vi "Write Controller Actor Enqueuer.vi"(8 "error in (no error)":errorcluster, 10 "Controller Actor Enqueuer":refnum<class "Message Enqueuer.lvclass">, 11 "View Actor in":refnum<class "View Actor.lvclass">) -> (0 "error out":errorcluster, 3 "View Actor out":refnum<class "View Actor.lvclass">)   [LabVIEW 2016, in "Event Actors.lvlib" / "View Actor.lvclass"]
uses:
  View Actor.lvclass
  <vilib>/ActorFramework/Message Enqueuer/Message Enqueuer.lvclass
  View Actor.lvclass/View Actor.ctl
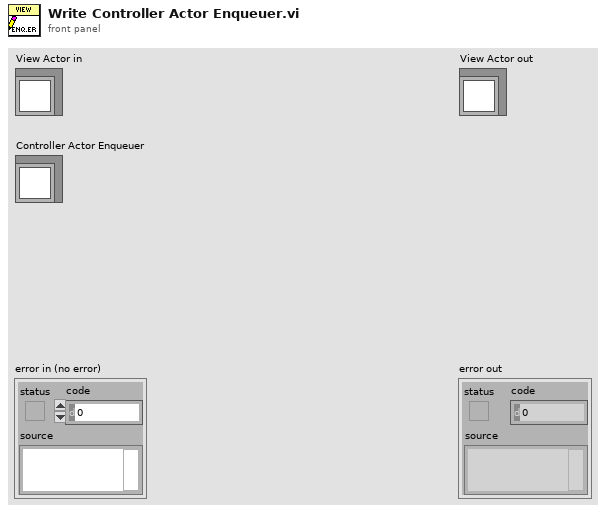
[diagram p1: front panel]
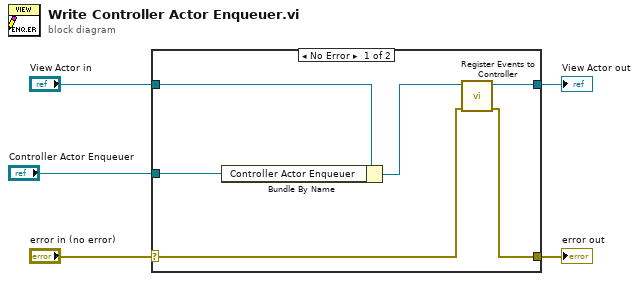
[diagram p0: block diagram]
diagram:
  n1 = case shown="No Error" "error in (no error)" {
    selector: "error in (no error)" -> [w7 w12]
    tunnel: [w6 w12] -> w4
    tunnel: [w8 w13] -> w2
    tunnel: "View Actor in" -> [w11 w13]
    tunnel: "Controller Actor Enqueuer" -> [w10 _]
    frame No Error {
      n2 = Bundle By Name(cluster=w11, "Controller Actor Enqueuer"=w10) -> (w9:refnum<class "View Actor.lvclass">)
      n3 = call-dynamic "Register Events to Controller.vi"("error in (no error)"=w7, "View Actor in"=w9) -> ("error out"=w6:errorcluster, "View Actor out"=w8:refnum<class "View Actor.lvclass">)  [unwired: 8 in]
    }
    frame Error {
    }
  }
  "error out" <- w4
  "View Actor out" <- w2
